vi "Init.vi"(10 "Data":T1) -> (3 "TEMPLATE Msg Contents out":refnum<class "TEMPLATE Msg Contents.lvclass">)   [LabVIEW 2020, in "_Template.lvlib" / "Templates.lvlib" / "TEMPLATE jettl Msg.lvlib" / "TEMPLATE Msg Contents.lvclass"]
uses:
  TEMPLATE Msg Contents.lvclass
  TEMPLATE Msg Contents.lvclass/TEMPLATE Msg Contents.ctl
  Data.ctl
  TEMPLATE jettl Msg.lvlib
panel:
  # "This front panel should not be manipulated."
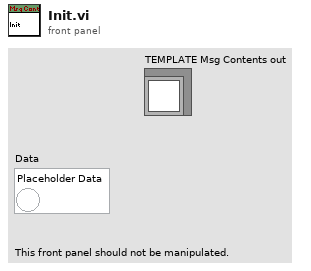
[diagram p1: front panel]
types:
  T1 = typedef "_Template.lvlib/Templates.lvlib/TEMPLATE jettl Msg.lvlib/Data.ctl" = cluster{"Placeholder Data":bool}
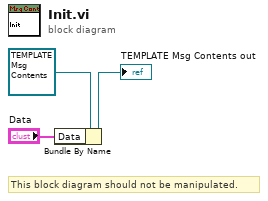
[diagram p0: block diagram]
diagram:
  # "This block diagram should not be manipulated."
  n1 = Bundle By Name(cluster=refnum<class "TEMPLATE Msg Contents.lvclass"> refnum ("_Template.lvlib:Templates.lvlib:TEMPLATE jettl Msg.lvlib:TEMPLATE Msg Input.lvclass"), "Data"="Data") -> (→"TEMPLATE Msg Contents out":refnum<class "TEMPLATE Msg Contents.lvclass">)
